vi "Add shift register.vi"(0 "Loop Reference":refnum<vi>, 1 "Right Outside Terminal Sink":refnum<vi>, 5 "Right Inside Terminal Source":refnum<vi>, 9 "Left Outside Terminal Source":refnum<vi>, 11 "error in (no error)":errorcluster, 12 "Left Inside Terminal Sink":refnum<vi>, 13 "Y Positon":u32) -> (2 "New Shift Register":refnum<vi>, 3 "Right Inside Terminal":refnum<vi>, 4 "Loop ReferenceOut":refnum<vi>, 6 "Right Outside Terminal":refnum<vi>, 10 "Left Inside Terminal":refnum<vi>, 14 "Left Outside Terminal":refnum<vi>, 15 "error out":errorcluster)   [LabVIEW 2018, in "Scripting Tools.lvlib"]
doc: "Adds a shift register to the G Loop object and wires it up to the specified sources and sinks. Returns references to the shift register object, and the terminals that are wire sources (outputs)."
uses:
  Scripting Tools.lvlib
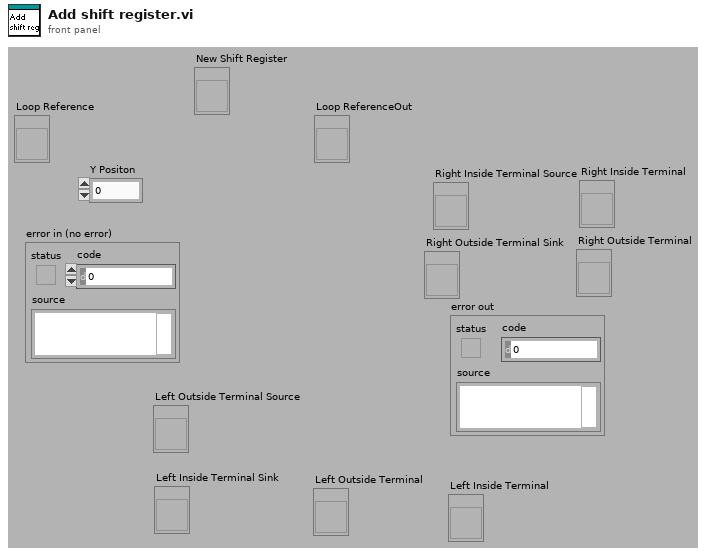
[diagram p1: front panel]
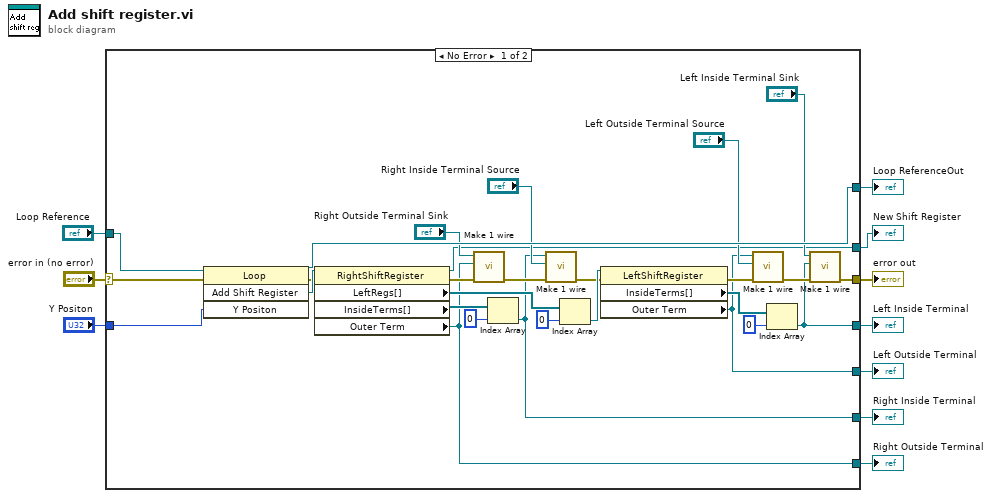
[diagram p0: block diagram]
diagram:
  n1 = case shown="No Error" "error in (no error)" {
    selector: "error in (no error)" -> [w11 w39]
    tunnel: "Loop Reference" -> [w38 _]
    tunnel: [w37 _] -> w9
    tunnel: "Y Positon" -> [w36 _]
    tunnel: [w21 w39] -> w7
    tunnel: [w19 _] -> w6
    tunnel: [w17 _] -> w5
    tunnel: [w16 _] -> w4
    tunnel: [w13 _] -> w3
    tunnel: [w12 _] -> w2
    frame No Error {
      n2 = invoke on="Invoke Node" class="Loop" method="Add Shift Register"(reference=w38, error in=w11, "Y Positon"=w36) -> (reference out=w37:refnum<vi>, error out=w34:errorcluster, "Add Shift Register"=w35:refnum<vi>)  [unwired: 1 in, 1 out]
      n3 = property on="Property Node" class="RightShiftRegister"(reference=w35, error in=w34) -> (reference out=w12:refnum<vi>, error out=w33:errorcluster, "LeftRegs[]"=w29:refnum<vi>[], "InsideTerms[]"=w32:refnum<vi>[], "Outer Term"=w16:refnum<vi>)
      n4 = call "Make 1 wire.vi"("error in"=w33, "Wire Terminal 2"=w16, "Wire Terminal 1"="Right Outside Terminal Sink") -> ("error out"=w30:errorcluster)  [unwired: 8 out]
      n5 = Index Array(array=w32, index=0) -> (element=w13:refnum<vi>)
      n6 = call "Make 1 wire.vi"("error in"=w30, "Wire Terminal 2"="Right Inside Terminal Source", "Wire Terminal 1"=w13) -> ("error out"=w26:errorcluster)  [unwired: 8 out]
      n7 = Index Array(array=w29, index=0) -> (element=w27:refnum<vi>)
      n8 = property on="Property Node" class="LeftShiftRegister"(reference=w27, error in=w26) -> (error out=w25:errorcluster, "InsideTerms[]"=w24:refnum<vi>[], "Outer Term"=w19:refnum<vi>)  [unwired: 1 out]
      n9 = call "Make 1 wire.vi"("error in"=w25, "Wire Terminal 2"="Left Outside Terminal Source", "Wire Terminal 1"=w19) -> ("error out"=w22:errorcluster)  [unwired: 8 out]
      n10 = Index Array(array=w24, index=0) -> (element=w17:refnum<vi>)
      n11 = call "Make 1 wire.vi"("error in"=w22, "Wire Terminal 2"=w17, "Wire Terminal 1"="Left Inside Terminal Sink") -> ("error out"=w21:errorcluster)  [unwired: 8 out]
    }
    frame Error {
    }
  }
  "Loop ReferenceOut" <- w9
  "Right Outside Terminal" <- w4
  "Right Inside Terminal" <- w3
  "Left Outside Terminal" <- w6
  "Left Inside Terminal" <- w5
  "error out" <- w7
  "New Shift Register" <- w2
